vi "Translate into Cluster Element.vi"(8 "error in":errorcluster, 11 "LVData":refnum<class "variant.lvclass">) -> (0 "error out":errorcluster, 3 "LVData outs":refnum<class "variant.lvclass">)   [LabVIEW 2020, in "variant.lvlib" / "variant.lvclass"]
doc: "Returns the data names of the cluster elements."
uses:
  variant.lvclass
  Type Descriptor/TD.lvclass
panel:
  in  "element":i32
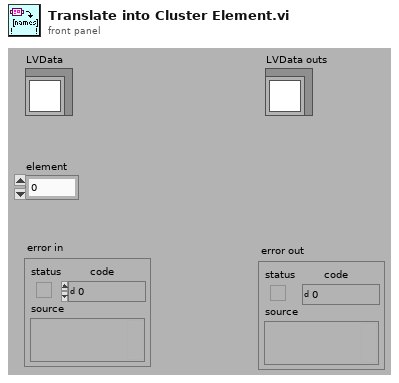
[diagram p1: front panel]
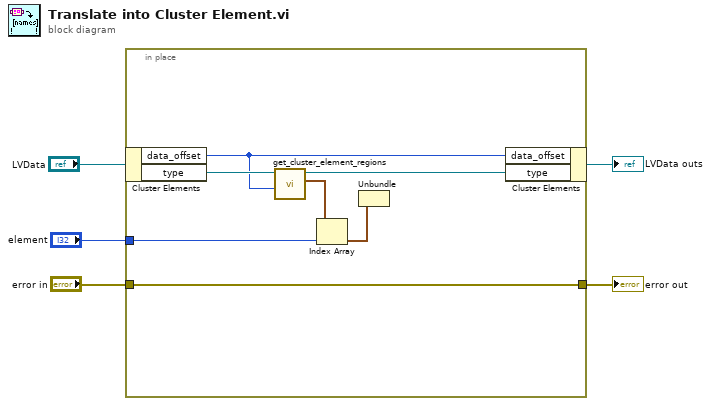
[diagram p0: block diagram]
diagram:
  n1 = in-place {
    in-place-border: [w10] -> w3
    in-place-border: "error in" -> [w10]
    in-place-border: "element" -> [w8]
    n2 = in-place-cluster #1("LVData") -> ("data_offset"=w6:i32, "type"=w12:refnum<class "TD.lvclass">)
    n3 = call "get_cluster_element_regions.vi"("cluster offset"=w6, "TypeDescriptor"=w12) -> ("element_regions"=w9:cluster{i32, i32}[], "TypeDescriptor out"=w11:refnum<class "TD.lvclass">)  [unwired: 7 in, 1 out]
    n4 = Index Array(array=w9, index=w8) -> (element=w7:cluster{i32, i32})
    n5 = Unbundle(w7) -> ()  [unwired: 2 out]
    n6 = in-place-cluster #1("data_offset"=w6, "type"=w11) -> (→"LVData outs":refnum<class "variant.lvclass">)
  }
  "error out" <- w3
